vi "Initialize Sessions - NSess.vi"(6 "initialize and close session behavior":T1, 8 "error in":errorcluster, 11 "session reservation in":refnum<class "Session Reservation.lvclass">) -> (0 "error out":errorcluster, 1 "channel lists":string[](array[string]), 2 "sessions":string[](array[string]), 3 "session reservation out":refnum<class "Session Reservation.lvclass">)   [LabVIEW 2025, in "Session Management seMultiplexer.lvlib"]
uses:
  Session Management seMultiplexer.lvlib
  b67e8fb3-ad6d-4d65-aece-693a4f0e2f78.vi
  Session Factory/Session Factory.lvclass
  <vilib>/Plug-In SDKs/Clients/Session Management V1/Session Reservation/Session Reservation.lvclass
  <vilib>/Plug-In SDKs/Clients/Session Management V1/Session Reservation/Initialize and Close Session Behavior.ctl
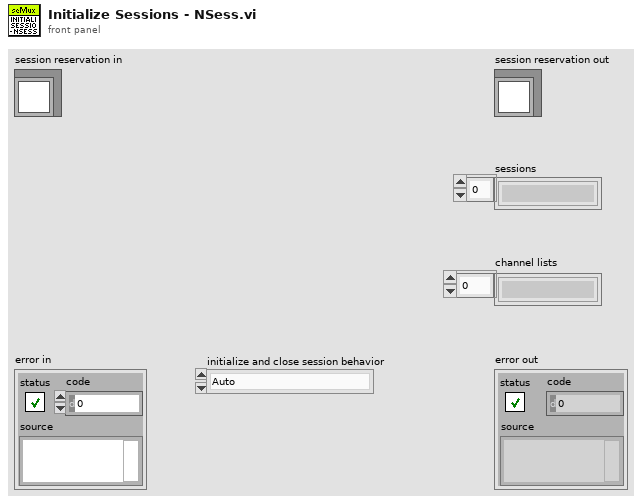
[diagram p1: front panel]
types:
  T1 = typedef "NI Session Management V1 Client.lvlib/Session Reservation.lvclass/Initialize and Close Session Behavior.ctl" = enum16{"Auto", "Initialize and Close", "Attach and Detach", "Initialize and Detach", "Attach and Close"}
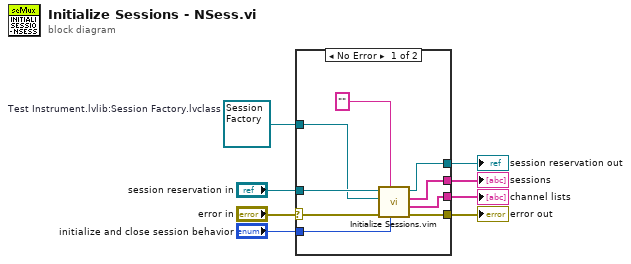
[diagram p0: block diagram]
diagram:
  w1 = refnum<class "Session Factory.lvclass"> refnum  # Test Instrument.lvlib:Session Factory.lvclass
  n1 = case shown="No Error" "error in" {
    selector: "error in" -> [w9 w19]
    tunnel: [w15 w19] -> w7
    tunnel: [w16 w18] -> w5
    tunnel: "session reservation in" -> [w17 w18]
    tunnel: [w14 _] -> w3
    tunnel: [w13 _] -> w4
    tunnel: "initialize and close session behavior" -> [w12 _]
    tunnel: w1 -> [w10 _]
    frame No Error {
      n2 = call "Initialize Sessions.vim"("initialize and close session behavior"=w12, "session type"="", "error in"=w9, "session factory"=w10, "session reservation in"=w17) -> ("error out"=w15:errorcluster, "channel lists"=w13:string[], "sessions"=w14:string[], "session reservation out"=w16:refnum<class "Session Reservation.lvclass">)  [unwired: 3 in]
    }
    frame Error {
    }
  }
  "error out" <- w7
  "session reservation out" <- w5
  "channel lists" <- w4
  "sessions" <- w3
